vi "Follow Aircraft.vi"(8 "Error In":errorcluster, 10 "Follow?":bool, 11 "Aircraft ID":u8) -> (0 "error out":errorcluster)   [LabVIEW 2014]
uses:
  Aircraft Information/Sub VI/Get Aircraft GPS.vi
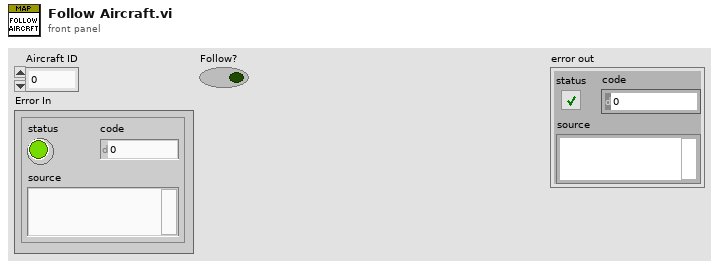
[diagram p1: front panel]
types:
  T1 = typedef "Aircraft GPS Data.ctl" = cluster{"Latitude (degrees)":dbl, "Longitude (degrees)":dbl, "Altitude (m)":dbl, "Fix Type":T2, "HDOP (cm)":u16, "VDOP (cm)":u16, "Ground Speed (m/s)":dbl, "Coarse Over Ground (degrees)":u16, "Number of Satellites":u8}
  T2 = typedef "GPS Fix Type.ctl" = enum16{"No Fix 0", "No Fix 1", "2D Fix", "3D Fix", "DGPS", "RTK"}
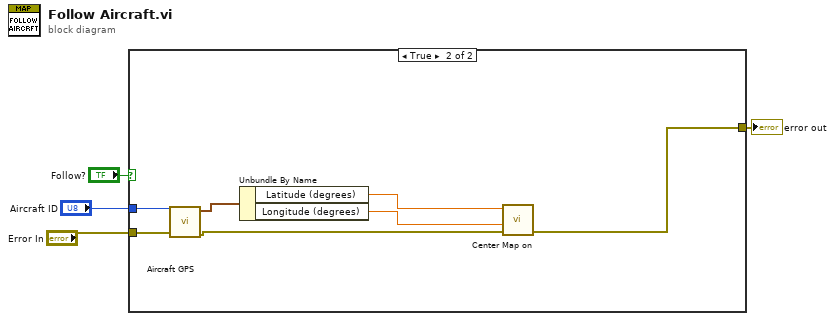
[diagram p0: block diagram]
diagram:
  n1 = case shown="True" "Follow?" {
    tunnel: "Aircraft ID" -> [_ w10]
    tunnel: "Error In" -> [w5 w9]
    tunnel: [w5 w6] -> w2
    frame False {
    }
    frame True {
      n2 = call-poly "Aircraft GPS.vi"("Error In"=w9, "Aircraft ID"=w10) -> ("Error Out"=w6:errorcluster, "Aircraft GPS Data Out"=w11:T1)  [unwired: 8 in]
      n3 = Unbundle By Name(w11) -> ("Latitude (degrees)"=w8:dbl, "Longitude (degrees)"=w7:dbl)
      n4 = call "Center Map on.vi"("lng"=w7, "lat"=w8) -> ()  [unwired: 9 in, 1 out]
    }
  }
  "error out" <- w2
